vi "UndotOrNot.vi"(9 "UnDot?":bool, 11 "DottedNumber":string) -> (1 "Number":dbl, 3 "result string":string)   [LabVIEW 2021, in "Files.lvlib"]
uses:
  Files.lvlib
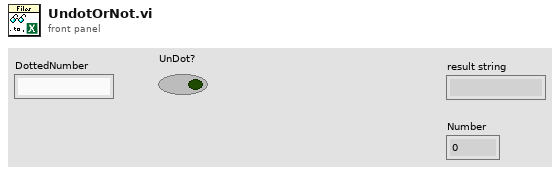
[diagram p1: front panel]
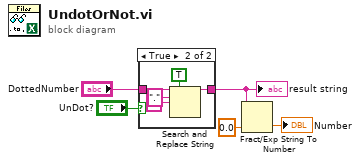
[diagram p0: block diagram]
diagram:
  n1 = case shown="True" "UnDot?" {
    tunnel: "DottedNumber" -> [w6 w11]
    tunnel: [w6 w10] -> w2
    frame False {
    }
    frame True {
      n2 = Search and Replace String(replace all?=TRUE ("replace all? (F)"), input string=w11, search string=".", replace string="," ("replace string (\"\")")) -> (result string=w10:string)  [unwired: 4 in, 3 out]
    }
  }
  "result string" <- w2
  n3 = Fract/Exp String To Number(string=w2, default (0 dbl)=0.0 ("default")) -> (number=→"Number":dbl)  [unwired: 2 in, 1 out]
